vi "DtCreateCtrEventsChan.vi"(5 "Board Name":string, 7 "Counter Num":u32, 9 "Gate Type":i32(ring)=2 items=["Low Level", "High Level", "None"], 11 "error in (no error)":errorcluster) -> (4 "Task out":i32, 15 "error out 2":errorcluster)   [LabVIEW 2022 SP3]
doc: "Creates one or more virtual counter/timer channels that count digital pulses from an external signal, which is connected to the counter/timer's clock input source, when the counter/timer is enabled (determined by the counter/timer's gate input signal)."
uses:
  DtLvLink.lvlib
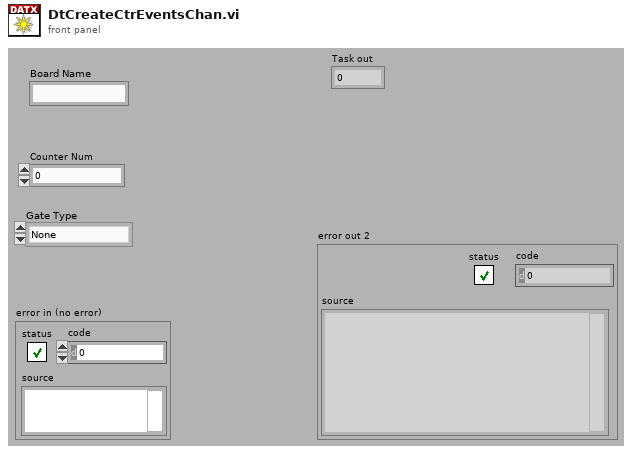
[diagram p1: front panel]
types:
  T1 = enum32{"AnalogInput", "AnalogOutput", "DigitalInput", "DigitalOutput", "Quadrature", "CounterTimer"}
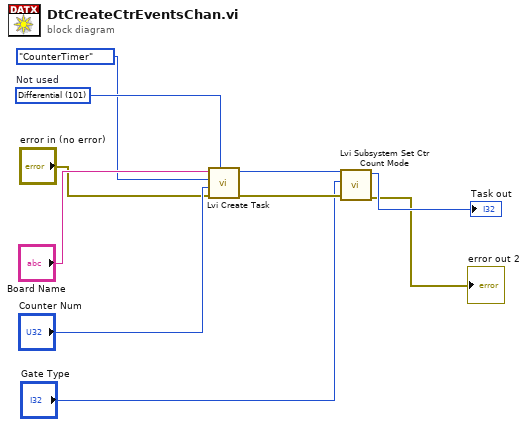
[diagram p0: block diagram]
diagram:
  w10 = 101 items=["SingleEnded"=100, "Differential"=101]  # Not used
  n1 = call "Lvi Create Task.vi"("SEorDiff"=w10, "error in (no error)"="error in (no error)", "SubSysIndex"="Counter Num", "ChanType"=T1."CounterTimer", "BoardName"="Board Name") -> ("error out"=w6:errorcluster, "TaskRef"=w5:i32)  [unwired: 4 in, 1 out]
  n2 = call "Lvi Subsystem Set Ctr Count Mode.vi"("error in (no error)"=w6, "GateLevel"="Gate Type", "TaskRef"=w5) -> ("error out"=→"error out 2":errorcluster, "TaskRef out"=→"Task out":i32)  [unwired: 6 in, 1 out]
